vi "Format Error Message.vi"(8 "error in":errorcluster, 10 "Line":string, 11 "Line Number":i32) -> (0 "error out":errorcluster, 3 "Error Message":string)   [LabVIEW 2023]
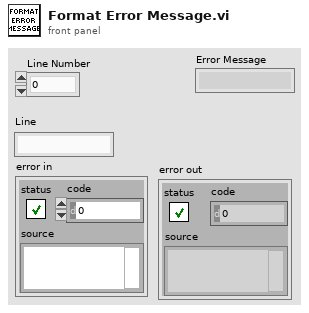
[diagram p1: front panel]
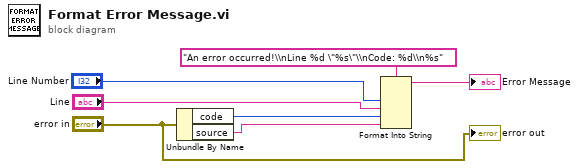
[diagram p0: block diagram]
diagram:
  n1 = Unbundle By Name("error in") -> ("code"=w3:i32, "source"=w2:string)
  n2 = Format Into String(format string="An error occurred!\\nLine %d \"%s\"\\nCode: %d\\n%s", "Line Number", "Line", w3, w2) -> (resulting string=→"Error Message":string)  [unwired: 2 in, 1 out]
  "error out" <- "error in"
